vi "ResonanceAnalyzer.vi"() -> ()   [LabVIEW 2015]
uses:
  <vilib>/imath/engines/lvmath2/RunTimeEngine/Managers/WorkSpace/UID Generator.vi
  <vilib>/imath/engines/lvmath2/RunTimeEngine/RunTimeType/NIMS_RunTimeType_From StrictType (excl LVString).vi
  <instcachedir>/0/NIMS_RunTimeType_From StrictType (excl LVString)_EB1C38A9BC5048DA9ABDA8F781E54D21.lvgen/NIMS_RunTimeType_From StrictType (excl LVString)_EB1C38A9BC5048DA9ABDA8F781E54D21_000.vi
  <vilib>/imath/engines/lvmath2/RunTimeEngine/LocalVariableDefStatement/MC_LocalVariableDefStatement_Display.vi
  <vilib>/imath/engines/lvmath2/RunTimeEngine/RangeToken/NIMS_Range.vi
  <instcachedir>/0/NIMS_Range_D919CC09935940E88F755EC1C6F49AC1.lvgen/NIMS_Range_D919CC09935940E88F755EC1C6F49AC1_000.vi
  <vilib>/imathl/engines/lvmath/Functions/Error Handling/Create Error.vi
  <vilib>/imath/engines/lvmath2/RunTimeEngine/BuiltInFunctions/randnormal/NIMS_randnormal(1,I32).vi
  <vilib>/imath/engines/lvmath2/RunTimeEngine/ErrorHandling/NIMS_Error From Error Code.vi
  <vilib>/imath/engines/lvmath2/RunTimeEngine/ArithmeticOperatorToken/NIMS_ArithmeticOperator_plus.vi
  <instcachedir>/0/NIMS_ArithmeticOperator_plus_A4F2756F5ADB4A0090E0DBD7C10701C8.lvgen/NIMS_ArithmeticOperator_plus_A4F2756F5ADB4A0090E0DBD7C10701C8_004.vi
  <vilib>/imath/engines/lvmath2/RunTimeEngine/Managers/SymbolTable/Clear UID.vi
  <vilib>/imath/engines/lvmath2/RunTimeEngine/NodeEndStatement/NIMS_NodeEndStatement_Output.vi
  <instcachedir>/0/NIMS_NodeEndStatement_Output_53EC0D466D134D7ABD903AC30B43404B.lvgen/NIMS_NodeEndStatement_Output_53EC0D466D134D7ABD903AC30B43404B_005.vi
  <vilib>/imath/engines/lvmath2/RunTimeEngine/ErrorHandling/NIMS_Finalize Error.vi
  <vilib>/Utility/file.llb/Read Delimited Spreadsheet (DBL).vi
  <vilib>/imath/engines/lvmath2/RunTimeEngine/Managers/SymbolTable/NIMS_WorkSpace.lvlib
panel:
  out "Results":T1={"Center Frequency"=600.0, "Amplitude"=1.0, "Q Factor"=10.0}
  out "XY Graph":cluster{"all rows":dbl[], "Array":dbl[]}[](graph)=[{"all rows"=[400.0, 405.0, 410.0, 415.0, 420.0, 425.0, 430.0, 435.0, 440.0, 445.0, 450.0, 455.0, 460.0, 465.0, 470.0, 475.0, 480.0, 485.0, 490.0, 495.0, 500.0, 505.0, 510.0, 515.0, 520.0, 525.0, 530.0, 535.0, 540.0, 545.0, 550.0, 555.0, 560.0, 565.0, 570.0, 575.0, 580.0, 585.0, 590.0, 595.0, 600.0, 605.0, 610.0, 615.0, 620.0, 625.0, 630.0, 635.0, 640.0, 645.0, 650.0, 655.0, 660.0, 665.0, 670.0, 675.0, 680.0, 685.0, 690.0, 695.0, 700.0, 705.0, 710.0, 715.0, 720.0, 725.0, 730.0, 735.0, 740.0, 745.0, 750.0, 755.0, 760.0, 765.0, 770.0, 775.0, 780.0, 785.0, 790.0, 795.0, 800.0], "Array"=[0.02200488997555012, 0.023121387283236993, 0.024324324324324322, 0.02562277580071174, 0.027027027027027025, 0.02854877081681205, 0.03020134228187919, 0.032, 0.033962264150943396, 0.03610832497492477, 0.03846153846153846, 0.041049030786773084, 0.04390243902439024, 0.047058823529411764, 0.05056179775280899, 0.05446293494704992, 0.0588235294117647, 0.06371681415929202, 0.06923076923076922, 0.07547169811320754, 0.08256880733944953, 0.0906801007556675, 0.09999999999999998, 0.11076923076923076, 0.12328767123287669, 0.13793103448275862, 0.15517241379310343, 0.17560975609756097, 0.19999999999999996, 0.22929936305732482, 0.2647058823529412, 0.30769230769230765, 0.36, 0.4235294117647058, 0.5, 0.5901639344262295, 0.6923076923076923, 0.7999999999999998, 0.9, 0.9729729729729728, 1.0, 0.9729729729729728, 0.9, 0.7999999999999998, 0.6923076923076923, 0.5901639344262295, 0.5, 0.4235294117647058, 0.36, 0.30769230769230765, 0.2647058823529412, 0.22929936305732482, 0.19999999999999996, 0.17560975609756097, 0.15517241379310343, 0.13793103448275862, 0.12328767123287669, 0.11076923076923076, 0.09999999999999998, 0.0906801007556675, 0.08256880733944953, 0.07547169811320754, 0.06923076923076922, 0.06371681415929202, 0.0588235294117647, 0.05446293494704992, 0.05056179775280899, 0.047058823529411764, 0.04390243902439024, 0.041049030786773084, 0.03846153846153846, 0.03610832497492477, 0.033962264150943396, 0.032, 0.03020134228187919, 0.02854877081681205, 0.027027027027027025, 0.02562277580071174, 0.024324324324324322, 0.023121387283236993, 0.02200488997555012]}, {"all rows"=[400.0, 405.0, 410.0, 415.0, 420.0, 425.0, 430.0, 435.0, 440.0, 445.0, 450.0, 455.0, 460.0, 465.0, 470.0, 475.0, 480.0, 485.0, 490.0, 495.0, 500.0, 505.0, 510.0, 515.0, 520.0, 525.0, 530.0, 535.0, 540.0, 545.0, 550.0, 555.0, 560.0, 565.0, 570.0, 575.0, 580.0, 585.0, 590.0, 595.0, 600.0, 605.0, 610.0, 615.0, 620.0, 625.0, 630.0, 635.0, 640.0, 645.0, 650.0, 655.0, 660.0, 665.0, 670.0, 675.0, 680.0, 685.0, 690.0, 695.0, 700.0, 705.0, 710.0, 715.0, 720.0, 725.0, 730.0, 735.0, 740.0, 745.0, 750.0, 755.0, 760.0, 765.0, 770.0, 775.0, 780.0, 785.0, 790.0, 795.0, 800.0], "Array"=[0.02200488997555012, 0.023121387283236993, 0.024324324324324322, 0.02562277580071174, 0.027027027027027025, 0.02854877081681205, 0.03020134228187919, 0.032, 0.033962264150943396, 0.03610832497492477, 0.03846153846153846, 0.041049030786773084, 0.04390243902439024, 0.047058823529411764, 0.05056179775280899, 0.05446293494704992, 0.0588235294117647, 0.06371681415929202, 0.06923076923076922, 0.07547169811320754, 0.08256880733944953, 0.0906801007556675, 0.09999999999999998, 0.11076923076923076, 0.12328767123287669, 0.13793103448275862, 0.15517241379310343, 0.17560975609756097, 0.19999999999999996, 0.22929936305732482, 0.2647058823529412, 0.30769230769230765, 0.36, 0.4235294117647058, 0.5, 0.5901639344262295, 0.6923076923076923, 0.7999999999999998, 0.9, 0.9729729729729728, 1.0, 0.9729729729729728, 0.9, 0.7999999999999998, 0.6923076923076923, 0.5901639344262295, 0.5, 0.4235294117647058, 0.36, 0.30769230769230765, 0.2647058823529412, 0.22929936305732482, 0.19999999999999996, 0.17560975609756097, 0.15517241379310343, 0.13793103448275862, 0.12328767123287669, 0.11076923076923076, 0.09999999999999998, 0.0906801007556675, 0.08256880733944953, 0.07547169811320754, 0.06923076923076922, 0.06371681415929202, 0.0588235294117647, 0.05446293494704992, 0.05056179775280899, 0.047058823529411764, 0.04390243902439024, 0.041049030786773084, 0.03846153846153846, 0.03610832497492477, 0.033962264150943396, 0.032, 0.03020134228187919, 0.02854877081681205, 0.027027027027027025, 0.02562277580071174, 0.024324324324324322, 0.023121387283236993, 0.02200488997555012]}]
  in  "Tab Control":enum32{"Simulation", "Experiment"}(tab)
  in  "Q":dbl=10.0
  in  "Center Frequency":dbl=600.0
  in  "Start Frequency":dbl=400.0
  in  "End Frequency":dbl=800.0
  in  "df":dbl=5.0
  in  "Noise Level":dbl
  in  "file path (dialog if empty)":path=path "C:/Users/minor6th/Desktop/PHYS434/week5/week5/Peakdata"
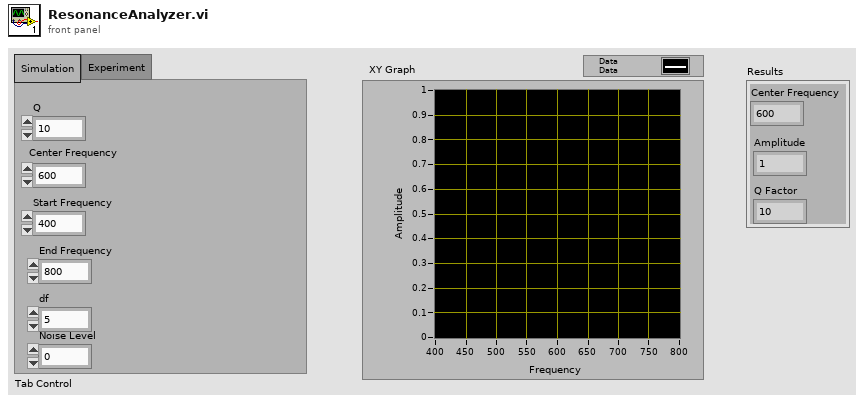
[diagram p1: front panel]
types:
  T1 = cluster{"Center Frequency":dbl, "Amplitude":dbl, "Q Factor":dbl}
  T2 = cluster{"Array[0]":dbl, "Array[1]":dbl, "Array[2]":dbl, "Array[3]":dbl, "Array[4]":dbl, "Array[5]":dbl, "Array[6]":dbl, "Array[7]":dbl, "Array[8]":dbl}
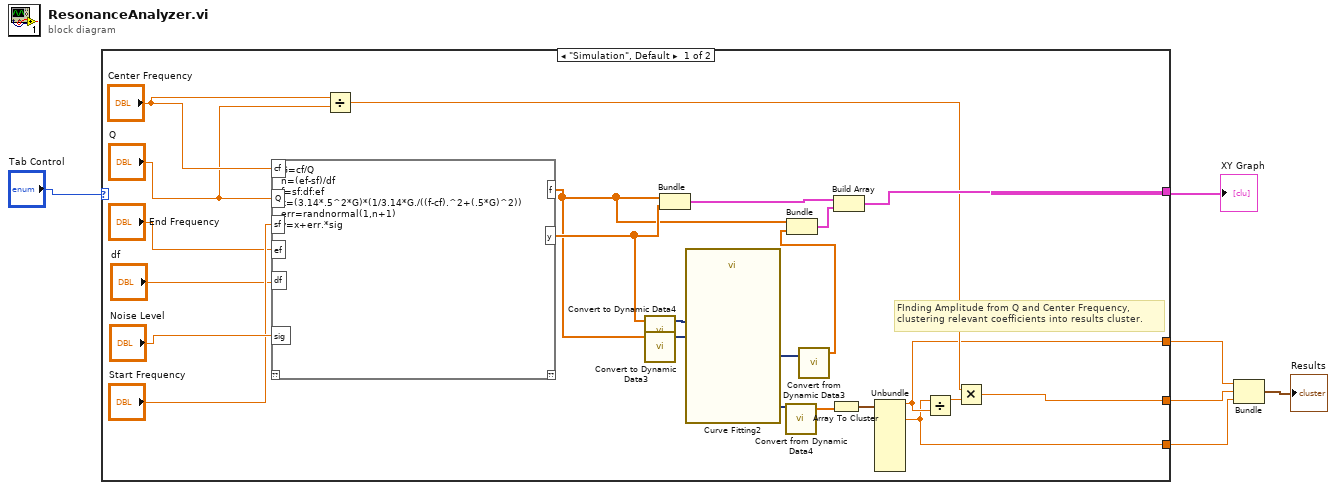
[diagram p0: block diagram]
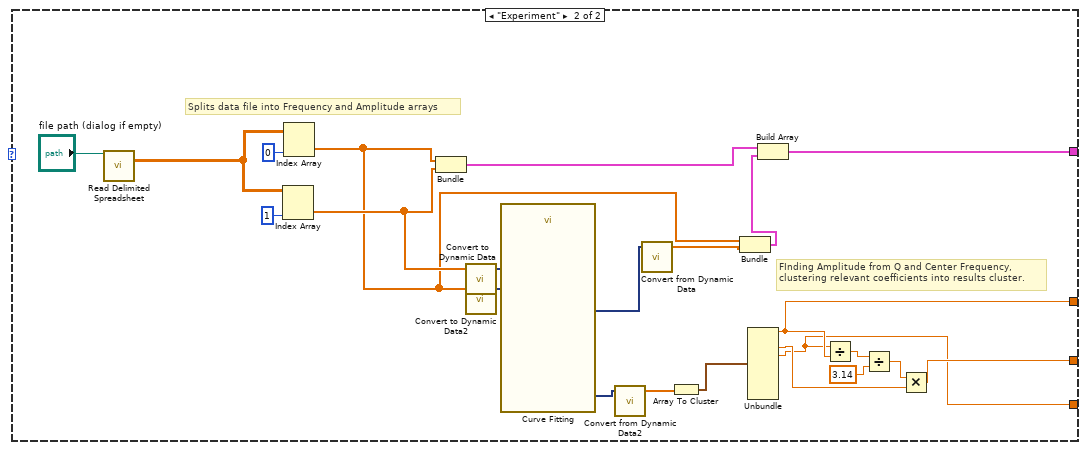
[diagram p2: hidden frame]
diagram:
  n1 = case shown="\"Simulation\", Default" "Tab Control" {
    tunnel: [w22 w221] -> w5
    tunnel: [w10 w214] -> w3
    tunnel: [w8 w213] -> w4
    tunnel: [w7 w212] -> w2
    frame "Simulation", Default {
      # "FInding Amplitude from Q and Center Frequency,\nclustering relevant coefficients into results cluster."
      n2 = mathscript code="G=cf/Q\nn=(ef-sf)/df\nf=sf:df:ef\nx=(3.14*.5^2*G)*(1/3.14*G./((f-cf).^2+(.5*G)^2))\nerr=randnormal(1,n+1)\ny=x+err.*sig"("sig"="Noise Level", "cf"="Center Frequency", "sf"="Start Frequency", "ef"="End Frequency", "df"="df", "Q"="Q") -> ("y"=w25:dbl[], "f"=w20:dbl[])  [unwired: 1 in, 1 out]
      n3 = Divide(x="Center Frequency", y="Q") -> (x/y=w9:dbl)
      n4 = call "Convert to Dynamic Data4"("Array"=w25) -> ("Dynamic Data Type"=w19:dynamicdata)  [unwired: 3 in]
      n5 = call "Convert to Dynamic Data3"("Array"=w20) -> ("Dynamic Data Type"=w18:dynamicdata)  [unwired: 3 in]
      n6 = Bundle("f"=w20, "y"=w25) -> (w24:cluster{"f":dbl[], "y":dbl[]})  [unwired: 1 in]
      n7 = call "Curve Fitting2"("Locations"=w18, "Signals"=w19) -> ("best fit"=w17:dynamicdata, "non-linear coefficients"=w16:dynamicdata)  [unwired: 5 in, 3 out]
      n8 = call "Convert from Dynamic Data4"("Dynamic Data Type"=w16) -> ("Array"=w15:dbl[])  [unwired: 3 in]
      n9 = call "Convert from Dynamic Data3"("Dynamic Data Type"=w17) -> ("Array"=w21:dbl[])  [unwired: 3 in]
      n10 = Bundle("f"=w20, "Array"=w21) -> (w23:cluster{"f":dbl[], "Array":dbl[]})  [unwired: 1 in]
      n11 = Array To Cluster(array=w15) -> (cluster=w14:T2)
      n12 = Build Array(w24, w23) -> (w22:cluster{"f":dbl[], "Array":dbl[]}[])
      n13 = Unbundle(w14) -> ("Array[0]"=w8:dbl, "Array[2]"=w7:dbl)  [unwired: 7 out]
      n14 = Divide(x=w7, y=w8) -> (x/y=w11:dbl)
      n15 = Multiply(x=w9, y=w11) -> (x*y=w10:dbl)
    }
    frame "Experiment" {
      # "Splits data file into Frequency and Amplitude arrays"
      # "FInding Amplitude from Q and Center Frequency,\nclustering relevant coefficients into results cluster."
      n16 = call-poly <vilib>:"Read Delimited Spreadsheet.vi"("file path (dialog if empty)"="file path (dialog if empty)") -> ("all rows"=w232:dbl[][])  [unwired: 9 in, 5 out]
      n17 = Index Array(array=w232, index (col)=1 ("disabled index (col)")) -> (element=w229:dbl[])  [unwired: 1 in]
      n18 = Index Array(array=w232, index (col)=0 ("disabled index (col)")) -> (element=w224:dbl[])  [unwired: 1 in]
      n19 = Bundle("all rows"=w224, "all rows"=w229) -> (w223:cluster{"all rows":dbl[], "all rows":dbl[]})  [unwired: 1 in]
      n20 = call "Convert to Dynamic Data"("Array"=w229) -> ("Dynamic Data Type"=w228:dynamicdata)  [unwired: 3 in]
      n21 = call "Convert to Dynamic Data2"("Array"=w224) -> ("Dynamic Data Type"=w227:dynamicdata)  [unwired: 3 in]
      n22 = call "Curve Fitting"("Locations"=w227, "Signals"=w228) -> ("best fit"=w226:dynamicdata, "non-linear coefficients"=w220:dynamicdata)  [unwired: 5 in, 3 out]
      n23 = call "Convert from Dynamic Data2"("Dynamic Data Type"=w220) -> ("Array"=w219:dbl[])  [unwired: 3 in]
      n24 = call "Convert from Dynamic Data"("Dynamic Data Type"=w226) -> ("Array"=w225:dbl[])  [unwired: 3 in]
      n25 = Array To Cluster(array=w219) -> (cluster=w211:T2)
      n26 = Bundle("all rows"=w224, "Array"=w225) -> (w222:cluster{"all rows":dbl[], "Array":dbl[]})  [unwired: 1 in]
      n27 = Unbundle(w211) -> ("Array[0]"=w213:dbl, "Array[2]"=w216:dbl, "Array[3]"=w212:dbl)  [unwired: 6 out]
      n28 = Build Array(w223, w222) -> (w221:cluster{"all rows":dbl[], "Array":dbl[]}[])
      n29 = Divide(x=w212, y=w213) -> (x/y=w218:dbl)
      n30 = Divide(x=w218, y=3.14) -> (x/y=w215:dbl)
      n31 = Multiply(x=w215, y=w216) -> (x*y=w214:dbl)
    }
  }
  "XY Graph" <- w5
  n32 = Bundle("Array[0]"=w4, w3, "Array[3]"=w2) -> (→"Results":cluster{"Array[0]":dbl, dbl, "Array[3]":dbl})  [unwired: 1 in]
